vi "Error.Display.vi"(8 "error in (no error)":errorcluster) -> ()   [LabVIEW 2015, in "Station.Execution.lvlib"]
uses:
  Station.Execution.lvlib
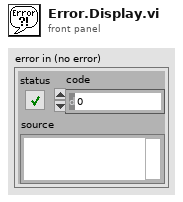
[diagram p1: front panel]
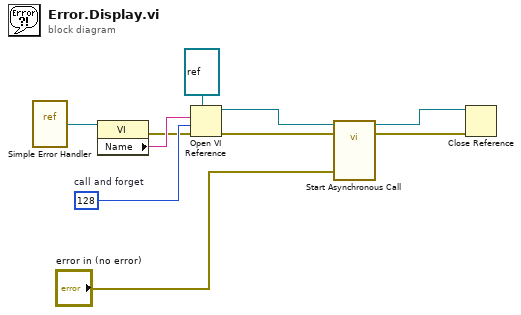
[diagram p0: block diagram]
diagram:
  w10 = 128  # call and forget
  n1 = vi-ref <vilib>:"Simple Error Handler.vi"() -> (w2:refnum<vi>)
  n2 = property class="VI"(reference=w2) -> (error out=w3:errorcluster, "Name"=w4:string)  [unwired: 1 in, 1 out]
  n3 = Open VI Reference(type specifier VI Refnum (for type only)=refnum<vi> refnum, vi path=w4, options=w10, error in (no error)=w3) -> (vi reference=w8:refnum<vi>, error out=w7:errorcluster)  [unwired: 2 in]
  n4 = call-by-ref "Start Asynchronous Call"(reference=w8, error in=w7, 9:"error in (no error)"="error in (no error)") -> (reference out=w5:refnum<vi>, error out=w6:errorcluster)  [unwired: 4 in, 5 out]
  n5 = Close Reference(reference=w5, error in (no error)=w6) -> ()  [unwired: 1 out]
